vi "HEWH RLT PRAT.vi"() -> ()   [LabVIEW 2016] (continued)
            n244 = Bundle("Core"=T66 {"Current VI Reference"=refnum, "Close Panel on Exit?"=FALSE}, "DrawsLeft"=w600, "Error Log"=w599, "RLT Station Channels"="RLT Station Channels", "Station A Display"="Station A Display", "Station B Display"="Station B Display", "Station C Display"="Station C Display", "Station D Display"="Station D Display", "Draw Parameters Seq"=T41 {"Draws Left"=0, "Draws Left Array"=[], "Remaining Draws (A)"=1000, "Remaining Draws (B)"=1000, "Remaining Draws (C)"=1000, "Remaining Draws (D)"=1000, "Index of Element (A-D)"=[], "Station A"={"Sequence #"=0.0, "Cycles"=0, "Mode Setting"="", "Flow Rate (GPM)"=0.0, "Temperature (F)"=0.0, "Reset Timer"=FALSE, "Use Temp Decline Method"=FALSE, "Terminate Condition"=enum."C1-Terminate Draw @ Gallon Mark", "Condition Value #1"=0.0, "UE"=FALSE, "LE"=FALSE, "Comp"=FALSE, "Fan"=FALSE, "Test End Time (Sec)"=0.0, "Purge Until Cutout"=FALSE, "Start Conditions"=enum."Heat Source Cutout", "Condition Value #2"=0.0, "Remove Power"=FALSE, "Time"=0.0, "Check Special Cond."=enum."SC2-Check Heat Source (On-C2/Off-C1)", "Condition#"=enum."C1", "Draw Flags"=enum."N/A", "Data Processing Delay (FHD 15sec, UEF 5 Sec)"=0.0, "Test Complete"=FALSE}, "Station B"={"Sequence #"=0.0, "Cycles"=0, "Mode Setting"="", "Flow Rate (GPM)"=0.0, "Temperature (F)"=0.0, "Reset Timer"=FALSE, "Use Temp Decline Method"=FALSE, "Terminate Condition"=enum."C1-Terminate Draw @ Gallon Mark", "Condition Value #1"=0.0, "UE"=FALSE, "LE"=FALSE, "Comp"=FALSE, "Fan"=FALSE, "Test End Time (Sec)"=0.0, "Purge Until Cutout"=FALSE, "Start Conditions"=enum."Heat Source Cutout", "Condition Value #2"=0.0, "Remove Power"=FALSE, "Time"=0.0, "Check Special Cond."=enum."SC2-Check Heat Source (On-C2/Off-C1)", "Condition#"=enum."C1", "Draw Flags"=enum."N/A", "Data Processing Delay (FHD 15sec, UEF 5 Sec)"=0.0, "Test Complete"=FALSE}, "Station C"={"Sequence #"=0.0, "Cycles"=0, "Mode Setting"="", "Flow Rate (GPM)"=0.0, "Temperature (F)"=0.0, "Reset Timer"=FALSE, "Use Temp Decline Method"=FALSE, "Terminate Condition"=enum."C1-Terminate Draw @ Gallon Mark", "Condition Value #1"=0.0, "UE"=FALSE, "LE"=FALSE, "Comp"=FALSE, "Fan"=FALSE, "Test End Time (Sec)"=0.0, "Purge Until Cutout"=FALSE, "Start Conditions"=enum."Heat Source Cutout", "Condition Value #2"=0.0, "Remove Power"=FALSE, "Time"=0.0, "Check Special Cond."=enum."SC2-Check Heat Source (On-C2/Off-C1)", "Condition#"=enum."C1", "Draw Flags"=enum."N/A", "Data Processing Delay (FHD 15sec, UEF 5 Sec)"=0.0, "Test Complete"=FALSE}, "Station D"={"Sequence #"=0.0, "Cycles"=0, "Mode Setting"="", "Flow Rate (GPM)"=0.0, "Temperature (F)"=0.0, "Reset Timer"=FALSE, "Use Temp Decline Method"=FALSE, "Terminate Condition"=enum."C1-Terminate Draw @ Gallon Mark", "Condition Value #1"=0.0, "UE"=FALSE, "LE"=FALSE, "Comp"=FALSE, "Fan"=FALSE, "Test End Time (Sec)"=0.0, "Purge Until Cutout"=FALSE, "Start Conditions"=enum."Heat Source Cutout", "Condition Value #2"=0.0, "Remove Power"=FALSE, "Time"=0.0, "Check Special Cond."=enum."SC2-Check Heat Source (On-C2/Off-C1)", "Condition#"=enum."C1", "Draw Flags"=enum."N/A", "Data Processing Delay (FHD 15sec, UEF 5 Sec)"=0.0, "Test Complete"=FALSE}}, "Current Cond A"=w591, "Current Cond B"=w590, "Current Cond C"=w589, "Current Cond D"=w588, "Power Analyzer"=w587) -> (w597:T70)  [unwired: 1 in]
          }
        }
        n245 = call <vilib>:"Add State(s) to Queue__jki_lib_state_machine.vi"("State(s) in (\"\")"=w586) -> ("States Out"=w585:string)  [unwired: 14 in]
      }
      frame "Data: Cleanup" {
        n246 = Unbundle By Name(w606) -> ("Core.Current VI Reference"=w605:refnum<vi>)
        n247 = Close Reference(reference=w605, error in (no error)=w604) -> (error out=w602:errorcluster)
        n248 = call <vilib>:"Add State(s) to Queue__jki_lib_state_machine.vi"("State(s) in (\"\")"=w608) -> ("States Out"=w607:string)  [unwired: 14 in]
      }
      frame "---------- UI ----------" {
        n249 = call <vilib>:"Add State(s) to Queue__jki_lib_state_machine.vi"("State(s) in (\"\")"=w613) -> ("States Out"=w612:string)  [unwired: 14 in]
      }
      frame "UI: Initialize" {
        w617 = FALSE ("Recording Data")
        n250 = local write "Init Complete"(w617) -> ()
        n251 = local write "Alarm A"(w617) -> ()
        n252 = local write "Alarm B"(w617) -> ()
        n253 = local write "Alarm C"(w617) -> ()
        n254 = local write "Alarm D"(w617) -> ()
        n255 = property on="Start/Pause test" class="Bool (strict)"("DisabledEnum"=T67."Disabled and Grayed Out" ("Disabled")) -> ()  [unwired: 2 in, 2 out]
        n256 = local read "LV Program"() -> (w615:T24)
        n257 = case shown="\"PRAT\"" w615 {
          frame "HEWH", Default {
            w625 = T67."Disabled and Grayed Out" ("Disabled")
            w638 = T67."Disabled and Grayed Out" ("Disabled")
            w639 = HEWH_RLT_Station_Disable."Disable Station (No Draw)" ("Disable Station 2")
            w640 = T67."Disabled and Grayed Out" ("Disabled")
            w643 = FALSE ("DAQ for B")
            w644 = T67."Disabled and Grayed Out" ("Disabled")
            w627 = T67."Disabled and Grayed Out" ("Disabled")
            w632 = T67."Disabled and Grayed Out" ("Disabled")
            w645 = T67."Enabled" ("Disabled")
            n258 = property on="IF Start" class="Bool"("DisabledEnum"=w645) -> ()  [unwired: 2 in, 2 out]
            n259 = property on="Inlet Valve A" class="CmbBox (strict)"("DisabledEnum"=T67."Enabled" ("Disabled")) -> (error out=w633:errorcluster)  [unwired: 2 in, 1 out]
            n260 = property on="Drain Valve A" class="CmbBox (strict)"("DisabledEnum"=T67."Enabled" ("Disabled")) -> (error out=w630:errorcluster)  [unwired: 2 in, 1 out]
            n261 = property on="Outlet Valve A" class="CmbBox (strict)"("DisabledEnum"=T67."Enabled" ("Disabled")) -> (error out=w624:errorcluster)  [unwired: 2 in, 1 out]
            n262 = property on="DAQ for A" class="Bool (strict)"("DisabledEnum"=T67."Enabled" ("Disabled")) -> ()  [unwired: 2 in, 2 out]
            n263 = property on="DAQ for B" class="Bool (strict)"("DisabledEnum"=w644) -> ()  [unwired: 2 in, 2 out]
            n264 = property on="Inlet Valve B" class="CmbBox (strict)"(error in=w633, "DisabledEnum"=w632) -> (error out=w635:errorcluster)  [unwired: 1 in, 1 out]
            n265 = property on="Drain Valve B" class="CmbBox (strict)"(error in=w630, "DisabledEnum"=w627) -> (error out=w629:errorcluster)  [unwired: 1 in, 1 out]
            n266 = property on="Outlet Valve B" class="CmbBox (strict)"(error in=w624, "DisabledEnum"=w625) -> (error out=w623:errorcluster)  [unwired: 1 in, 1 out]
            n267 = property on="IF Stop" class="Bool"("DisabledEnum"=w645) -> ()  [unwired: 2 in, 2 out]
            n268 = property on="DAQ for C" class="Bool (strict)"("DisabledEnum"=w644) -> ()  [unwired: 2 in, 2 out]
            n269 = property on="Inlet Valve C" class="CmbBox (strict)"(error in=w635, "DisabledEnum"=w632) -> (error out=w634:errorcluster)  [unwired: 1 in, 1 out]
            n270 = property on="Drain Valve C" class="CmbBox (strict)"(error in=w629, "DisabledEnum"=w627) -> (error out=w628:errorcluster)  [unwired: 1 in, 1 out]
            n271 = property on="Outlet Valve C" class="CmbBox (strict)"(error in=w623, "DisabledEnum"=w625) -> (error out=w622:errorcluster)  [unwired: 1 in, 1 out]
            n272 = property on="HEWH Power" class="Bool (strict)"("DisabledEnum"=w645) -> ()  [unwired: 2 in, 2 out]
            n273 = property on="DAQ for D" class="Bool (strict)"("DisabledEnum"=w644) -> ()  [unwired: 2 in, 2 out]
            n274 = property on="Inlet Valve D" class="CmbBox (strict)"(error in=w634, "DisabledEnum"=w632) -> ()  [unwired: 1 in, 2 out]
            n275 = property on="Drain Valve D" class="CmbBox (strict)"(error in=w628, "DisabledEnum"=w627) -> ()  [unwired: 1 in, 2 out]
            n276 = property on="Outlet Valve D" class="CmbBox (strict)"(error in=w622, "DisabledEnum"=w625) -> ()  [unwired: 1 in, 2 out]
            n277 = property on="Disable Station 2" class="Enum (strict)"("Value"=w639) -> ()  [unwired: 2 in, 2 out]
            n278 = property on="Disable Station 3" class="Enum (strict)"("Value"=w639) -> ()  [unwired: 2 in, 2 out]
            n279 = property on="Disable Station 4" class="Enum (strict)"("Value"=w639) -> ()  [unwired: 2 in, 2 out]
            n280 = property on="Trigger Draw B" class="Bool"("DisabledEnum"=w638) -> ()  [unwired: 2 in, 2 out]
            n281 = property on="Trigger Draw C" class="Bool"("DisabledEnum"=w638) -> ()  [unwired: 2 in, 2 out]
            n282 = property on="Trigger Draw D" class="Bool"("DisabledEnum"=w638) -> ()  [unwired: 2 in, 2 out]
            n283 = property on="Disable Station 1" class="Enum (strict)"("DisabledEnum"=T67."Enabled" ("Disabled")) -> ()  [unwired: 2 in, 2 out]
            n284 = property on="Disable Station 2" class="Enum (strict)"("DisabledEnum"=w640) -> ()  [unwired: 2 in, 2 out]
            n285 = property on="Disable Station 3" class="Enum (strict)"("DisabledEnum"=w640) -> ()  [unwired: 2 in, 2 out]
            n286 = property on="Disable Station 4" class="Enum (strict)"("DisabledEnum"=w640) -> ()  [unwired: 2 in, 2 out]
            n287 = property on="Trigger Draw A" class="Bool"("DisabledEnum"=T67."Enabled" ("Disabled")) -> ()  [unwired: 2 in, 2 out]
            n288 = local write "DAQ for A"(TRUE ("DAQ for A")) -> ()
            n289 = local write "DAQ for B"(w643) -> ()
            n290 = local write "DAQ for C"(w643) -> ()
            n291 = local write "DAQ for D"(w643) -> ()
          }
          frame "HEWH RLT" {
            w650 = T67."Enabled" ("Disabled")
            w652 = T67."Enabled" ("Disabled")
            w657 = T67."Enabled" ("Disabled")
            w662 = T67."Enabled" ("Disabled")
            w663 = T67."Enabled" ("Disabled")
            w664 = FALSE ("DAQ for B")
            w666 = T67."Enabled" ("Disabled")
            w665 = T67."Enabled" ("Disabled")
            n292 = property on="IF Start" class="Bool"("DisabledEnum"=w665) -> ()  [unwired: 2 in, 2 out]
            n293 = property on="Inlet Valve A" class="CmbBox (strict)"("DisabledEnum"=T67."Enabled" ("Disabled")) -> (error out=w658:errorcluster)  [unwired: 2 in, 1 out]
            n294 = property on="Drain Valve A" class="CmbBox (strict)"("DisabledEnum"=T67."Enabled" ("Disabled")) -> (error out=w655:errorcluster)  [unwired: 2 in, 1 out]
            n295 = property on="Outlet Valve A" class="CmbBox (strict)"("DisabledEnum"=T67."Enabled" ("Disabled")) -> (error out=w649:errorcluster)  [unwired: 2 in, 1 out]
            n296 = property on="DAQ for A" class="Bool (strict)"("DisabledEnum"=w666) -> ()  [unwired: 2 in, 2 out]
            n297 = property on="DAQ for B" class="Bool (strict)"("DisabledEnum"=w666) -> ()  [unwired: 2 in, 2 out]
            n298 = property on="Inlet Valve B" class="CmbBox (strict)"(error in=w658, "DisabledEnum"=w657) -> (error out=w660:errorcluster)  [unwired: 1 in, 1 out]
            n299 = property on="Drain Valve B" class="CmbBox (strict)"(error in=w655, "DisabledEnum"=w652) -> (error out=w654:errorcluster)  [unwired: 1 in, 1 out]
            n300 = property on="Outlet Valve B" class="CmbBox (strict)"(error in=w649, "DisabledEnum"=w650) -> (error out=w648:errorcluster)  [unwired: 1 in, 1 out]
            n301 = property on="IF Stop" class="Bool"("DisabledEnum"=w665) -> ()  [unwired: 2 in, 2 out]
            n302 = property on="DAQ for C" class="Bool (strict)"("DisabledEnum"=w666) -> ()  [unwired: 2 in, 2 out]
            n303 = property on="Inlet Valve C" class="CmbBox (strict)"(error in=w660, "DisabledEnum"=w657) -> (error out=w659:errorcluster)  [unwired: 1 in, 1 out]
            n304 = property on="Drain Valve C" class="CmbBox (strict)"(error in=w654, "DisabledEnum"=w652) -> (error out=w653:errorcluster)  [unwired: 1 in, 1 out]
            n305 = property on="Outlet Valve C" class="CmbBox (strict)"(error in=w648, "DisabledEnum"=w650) -> (error out=w647:errorcluster)  [unwired: 1 in, 1 out]
            n306 = property on="HEWH Power" class="Bool (strict)"("DisabledEnum"=w665) -> ()  [unwired: 2 in, 2 out]
            n307 = property on="DAQ for D" class="Bool (strict)"("DisabledEnum"=w666) -> ()  [unwired: 2 in, 2 out]
            n308 = property on="Inlet Valve D" class="CmbBox (strict)"(error in=w659, "DisabledEnum"=w657) -> ()  [unwired: 1 in, 2 out]
            n309 = property on="Drain Valve D" class="CmbBox (strict)"(error in=w653, "DisabledEnum"=w652) -> ()  [unwired: 1 in, 2 out]
            n310 = property on="Outlet Valve D" class="CmbBox (strict)"(error in=w647, "DisabledEnum"=w650) -> ()  [unwired: 1 in, 2 out]
            n311 = property on="Trigger Draw D" class="Bool"("DisabledEnum"=w662) -> ()  [unwired: 2 in, 2 out]
            n312 = property on="Trigger Draw C" class="Bool"("DisabledEnum"=w662) -> ()  [unwired: 2 in, 2 out]
            n313 = property on="Trigger Draw B" class="Bool"("DisabledEnum"=w662) -> ()  [unwired: 2 in, 2 out]
            n314 = property on="Trigger Draw A" class="Bool"("DisabledEnum"=w662) -> ()  [unwired: 2 in, 2 out]
            n315 = local write "DAQ for B"(w664) -> ()
            n316 = local write "DAQ for C"(w664) -> ()
            n317 = local write "DAQ for D"(w664) -> ()
            n318 = local write "DAQ for A"(w664) -> ()
            n319 = property on="Disable Station 1" class="Enum (strict)"("DisabledEnum"=w663) -> ()  [unwired: 2 in, 2 out]
            n320 = property on="Disable Station 2" class="Enum (strict)"("DisabledEnum"=w663) -> ()  [unwired: 2 in, 2 out]
            n321 = property on="Disable Station 3" class="Enum (strict)"("DisabledEnum"=w663) -> ()  [unwired: 2 in, 2 out]
            n322 = property on="Disable Station 4" class="Enum (strict)"("DisabledEnum"=w663) -> ()  [unwired: 2 in, 2 out]
          }
          frame "PRAT" {
            w670 = T67."Disabled and Grayed Out" ("Disabled")
            w672 = T67."Disabled and Grayed Out" ("Disabled")
            w677 = T67."Enabled" ("Disabled")
            w682 = T67."Enabled" ("Disabled")
            w683 = T67."Enabled" ("Disabled")
            w684 = FALSE ("DAQ for B")
            w686 = T67."Disabled and Grayed Out" ("Disabled")
            w685 = T67."Disabled and Grayed Out" ("Disabled")
            n323 = property on="Trigger Draw A" class="Bool"("DisabledEnum"=w682) -> ()  [unwired: 2 in, 2 out]
            n324 = property on="DAQ for A" class="Bool (strict)"("DisabledEnum"=w686) -> ()  [unwired: 2 in, 2 out]
            n325 = property on="IF Start" class="Bool"("DisabledEnum"=w685) -> ()  [unwired: 2 in, 2 out]
            n326 = property on="Trigger Draw B" class="Bool"("DisabledEnum"=w682) -> ()  [unwired: 2 in, 2 out]
            n327 = property on="Inlet Valve A" class="CmbBox (strict)"("DisabledEnum"=T67."Enabled" ("Disabled")) -> (error out=w678:errorcluster)  [unwired: 2 in, 1 out]
            n328 = property on="Drain Valve A" class="CmbBox (strict)"("DisabledEnum"=T67."Disabled and Grayed Out" ("Disabled")) -> (error out=w675:errorcluster)  [unwired: 2 in, 1 out]
            n329 = property on="Outlet Valve A" class="CmbBox (strict)"("DisabledEnum"=T67."Disabled and Grayed Out" ("Disabled")) -> (error out=w669:errorcluster)  [unwired: 2 in, 1 out]
            n330 = property on="DAQ for B" class="Bool (strict)"("DisabledEnum"=w686) -> ()  [unwired: 2 in, 2 out]
            n331 = property on="IF Stop" class="Bool"("DisabledEnum"=w685) -> ()  [unwired: 2 in, 2 out]
            n332 = property on="Trigger Draw C" class="Bool"("DisabledEnum"=w682) -> ()  [unwired: 2 in, 2 out]
            n333 = property on="DAQ for C" class="Bool (strict)"("DisabledEnum"=w686) -> ()  [unwired: 2 in, 2 out]
            n334 = property on="Inlet Valve B" class="CmbBox (strict)"(error in=w678, "DisabledEnum"=w677) -> (error out=w680:errorcluster)  [unwired: 1 in, 1 out]
            n335 = property on="Drain Valve B" class="CmbBox (strict)"(error in=w675, "DisabledEnum"=w672) -> (error out=w674:errorcluster)  [unwired: 1 in, 1 out]
            n336 = property on="Outlet Valve B" class="CmbBox (strict)"(error in=w669, "DisabledEnum"=w670) -> (error out=w668:errorcluster)  [unwired: 1 in, 1 out]
            n337 = property on="HEWH Power" class="Bool (strict)"("DisabledEnum"=w685) -> ()  [unwired: 2 in, 2 out]
            n338 = property on="DAQ for D" class="Bool (strict)"("DisabledEnum"=w686) -> ()  [unwired: 2 in, 2 out]
            n339 = property on="Trigger Draw D" class="Bool"("DisabledEnum"=w682) -> ()  [unwired: 2 in, 2 out]
            n340 = property on="Inlet Valve C" class="CmbBox (strict)"(error in=w680, "DisabledEnum"=w677) -> (error out=w679:errorcluster)  [unwired: 1 in, 1 out]
            n341 = property on="Drain Valve C" class="CmbBox (strict)"(error in=w674, "DisabledEnum"=w672) -> (error out=w673:errorcluster)  [unwired: 1 in, 1 out]
            n342 = property on="Outlet Valve C" class="CmbBox (strict)"(error in=w668, "DisabledEnum"=w670) -> (error out=w667:errorcluster)  [unwired: 1 in, 1 out]
            n343 = property on="Inlet Valve D" class="CmbBox (strict)"(error in=w679, "DisabledEnum"=w677) -> ()  [unwired: 1 in, 2 out]
            n344 = property on="Drain Valve D" class="CmbBox (strict)"(error in=w673, "DisabledEnum"=w672) -> ()  [unwired: 1 in, 2 out]
            n345 = property on="Outlet Valve D" class="CmbBox (strict)"(error in=w667, "DisabledEnum"=w670) -> ()  [unwired: 1 in, 2 out]
            n346 = local write "DAQ for B"(w684) -> ()
            n347 = local write "DAQ for C"(w684) -> ()
            n348 = local write "DAQ for D"(w684) -> ()
            n349 = local write "DAQ for A"(w684) -> ()
            n350 = property on="Disable Station 1" class="Enum (strict)"("DisabledEnum"=w683) -> ()  [unwired: 2 in, 2 out]
            n351 = property on="Disable Station 2" class="Enum (strict)"("DisabledEnum"=w683) -> ()  [unwired: 2 in, 2 out]
            n352 = property on="Disable Station 3" class="Enum (strict)"("DisabledEnum"=w683) -> ()  [unwired: 2 in, 2 out]
            n353 = property on="Disable Station 4" class="Enum (strict)"("DisabledEnum"=w683) -> ()  [unwired: 2 in, 2 out]
          }
        }
        n354 = call <vilib>:"Add State(s) to Queue__jki_lib_state_machine.vi"("State(s) in (\"\")"=w621) -> ("States Out"=w620:string)  [unwired: 14 in]
      }
      frame "UI: Cursor Set" {
        # "Argument"
        # "Set and Unset Cursor Busy.\n(Usage: \"UI: Cursor Set >> Busy|Idle\")"
        n355 = case shown="\"Busy\"" w688 {
          tunnel: w690 -> [w695 w697]
          tunnel: [w694 w696] -> w689
          frame "Idle", Default {
            n356 = call <vilib>:"Unset Busy.vi"("error in (no error)"=w695) -> ("error out"=w694:errorcluster)  [unwired: 10 in]
          }
          frame "Busy" {
            n357 = call <vilib>:"Set Busy.vi"("error in (no error)"=w697) -> ("error out"=w696:errorcluster)  [unwired: 9 in, 1 out]
          }
        }
        n358 = call <vilib>:"Add State(s) to Queue__jki_lib_state_machine.vi"("State(s) in (\"\")"=w693) -> ("States Out"=w692:string)  [unwired: 14 in]
      }
      frame "UI: Front Panel State" {
        # "Argument"
        n359 = Unbundle By Name(w701) -> ("Core.Current VI Reference"=w700:refnum<vi>)
        n360 = case shown="\"Open\", Default" w699 {
          tunnel: w703 -> [w709 w722]
          tunnel: [w711 w723] -> w702
          tunnel: w700 -> [w710 w720]
          frame "Open", Default {
            n361 = property class="VI"(reference=w710, error in=w709) -> (reference out=w707:refnum<vi>, error out=w708:errorcluster, "Front Panel.Open"=w706:bool)
            n362 = case shown="False" w706 {
              tunnel: [w714 w717] -> w711
              tunnel: w708 -> [w713 w717]
              tunnel: w707 -> [w712 _]
              frame False {
                n363 = invoke class="VI" method="FP.Open"(reference=w712, error in=w713, "Activate"=TRUE, "State"=T68."Maximized") -> (error out=w714:errorcluster)  [unwired: 1 in, 4 out]
              }
              frame True {
              }
            }
          }
          frame "Close" {
            n364 = property class="VI"(reference=w720, error in=w722) -> (reference out=w719:refnum<vi>, error out=w721:errorcluster, "Front Panel.Open"=w718:bool)
            n365 = case shown="False" w718 {
              tunnel: [w724 w727] -> w723
              tunnel: w721 -> [w724 w726]
              tunnel: w719 -> [_ w725]
              frame False {
              }
              frame True {
                n366 = disable-structure shown="Enabled" {
                  disable-tunnel: [w730 w731] -> w727
                  disable-tunnel: w726 -> [w729 w731]
                  disable-tunnel: w725 -> [w728 _]
                  frame Disabled {
                    n367 = invoke class="VI" method="FP.Close"(reference=w728, error in=w729) -> (error out=w730:errorcluster)  [unwired: 1 in, 2 out]
                  }
                  frame Enabled {
                  }
                }
              }
            }
          }
        }
        n368 = call <vilib>:"Add State(s) to Queue__jki_lib_state_machine.vi"("State(s) in (\"\")"=w705) -> ("States Out"=w704:string)  [unwired: 14 in]
      }
      frame "---------- Macro ----------" {
        n369 = call <vilib>:"Add State(s) to Queue__jki_lib_state_machine.vi"("State(s) in (\"\")"=w736) -> ("States Out"=w735:string)  [unwired: 14 in]
      }
      frame "Macro: Initialize" {
        w738 = "Data: Initialize\nInitialize Core Data\nUI: Initialize\nUI: Front Panel State >> Open\nInitialize Channels\nInitialize Files\nTest: Update Display A\nTest: Update Display B\nTest: Update Display C\nTest: Update Display D\nInit Complete"  # Data: Initialize Initialize Core Data UI: Initialize UI: Front Panel State >> Open Initialize Channels Initialize Files Test: Update Display A Test: Update Display B Test: Update Display C Test: Update Display D Init Complete
        n370 = call <vilib>:"Add State(s) to Queue__jki_lib_state_machine.vi"("State(s) in Front (\"\")"=w738, "State(s) in (\"\")"=w742) -> ("States Out"=w741:string)  [unwired: 13 in]
      }
      frame "Macro: Exit" {
        n371 = Unbundle By Name(w750) -> ("Core.Close Panel on Exit?"=w749:bool)
        n372 = Select(t="UI: Front Panel State >> Close", s=w749, f="") -> (s? t:f=w746:string)
        n373 = call <vilib>:"Add State(s) to Queue__jki_lib_state_machine.vi"("State(s) in (\"\")"=w746, "State(s) at Back (\"\")"="Data: Cleanup\nExit") -> ("States Out"=w744:string)  [unwired: 13 in]
        n374 = call <vilib>:"Add State(s) to Queue__jki_lib_state_machine.vi"("State(s) in Front (\"\")"=w744, "State(s) in (\"\")"=w753) -> ("States Out"=w752:string)  [unwired: 13 in]
      }
      frame "---------- Test ----------" {
        n375 = call <vilib>:"Add State(s) to Queue__jki_lib_state_machine.vi"("State(s) in (\"\")"=w758) -> ("States Out"=w757:string)  [unwired: 14 in]
      }
      frame "Test: Check Complete" {
        n376 = Unbundle By Name(w788) -> ("Station A Display.Display Data (RLT).Cycle Count Display"=w780:i32, "Station A Display.Display Data (RLT).Cycle Count Display"=w781:i32, "Station A Display.Display Data (RLT).Cycle Count Display"=w782:i32, "Station A Display.Display Data (RLT).Cycle Count Display"=w783:i32)
        n377 = local read "Station A Test Sequence"() -> (w787:T14[])
        n378 = local read "Station B Test Sequence"() -> (w786:T14[])
        n379 = local read "Station C Test Sequence"() -> (w785:T14[])
        n380 = local read "Station D Test Sequence"() -> (w784:T14[])
        n381 = local read "Use Last Start Condition A?"() -> (w774:bool)
        n382 = local read "Use Last Start Condition B?"() -> (w773:bool)
        n383 = local read "Use Last Start Condition C?"() -> (w772:bool)
        n384 = local read "Use Last Start Condition D?"() -> (w771:bool)
        n385 = call "PRAT Multi Station Check.vi"("Station A Test Sequence"=w787, "Station B Test Sequence"=w786, "Station C Test Sequence"=w785, "Station D Test Sequence"=w784, "Error In"=w779, "Cycle Count Display (Station A)"=w783, "Use Last Start Condition A?"=w774, "Cycle Count Display (Station B)"=w782, "Cycle Count Display (Station C)"=w781, "Use Last Start Condition B?"=w773, "Cycle Count Display (Station D)"=w780, "Use Last Start Condition C?"=w772, "Use Last Start Condition D?"=w771) -> ("Draw Parameters"=w770:T41, "Error Out"=w761:errorcluster)  [unwired: 13 in]
        "Current Draw Parameters" <- w770
        n386 = Unbundle By Name(w770) -> ("Remaining Draws (A)"=→"Remaining Draws (A)":i32, "Remaining Draws (B)"=→"Remaining Draws (B)":i32, "Remaining Draws (C)"=→"Remaining Draws (C)":i32, "Remaining Draws (D)"=→"Remaining Draws (D)":i32, "Draws Left"=w769:i32)
        "Draws Left" <- w769
        n387 = local read "Log Data Output (D)"() -> (w766:bool)
        n388 = local read "Log Data Output (C)"() -> (w765:bool)
        n389 = local read "LV Program"() -> (w762:T24)
        n390 = local read "Log Data Output (A)"() -> (w768:bool)
        n391 = local read "Log Data Output (B)"() -> (w767:bool)
        n392 = call "HEWH Create Save Data States.vi"("LV Program"=w762, "Data Loop?"=FALSE, "Error In"=w761, "Log Data Output (C)"=w765, "Log Data Output (A)"=w768, "Log Data Output (D)"=w766, "Log Data Output (B)"=w767) -> ("SM States"=w763:string, "Error Out"=w760:errorcluster)  [unwired: 11 in]
        n393 = case shown="0" w769 {
          tunnel: w760 -> [w794 w798]
          tunnel: [w793 w798] -> w759
          frame 0 {
            n394 = call "UTILITY String Notifier.vi"("Status"=UTILITY_Notifier."Set", "error in (no error)"=w794, "Set Status"=T7 "All Draws Complete..." ("Message"), "name (unnamed)"="Message") -> ("error out"=w793:errorcluster)  [unwired: 6 in, 1 out]
          }
          frame 1, Default {
          }
        }
        n395 = Bundle By Name(cluster=w788, "Draw Parameters Seq"=w770) -> (w790:T70)
        n396 = call <vilib>:"Add State(s) to Queue__jki_lib_state_machine.vi"("State(s) in Front (\"\")"=w763, "State(s) in (\"\")"=w792) -> ("States Out"=w791:string)  [unwired: 13 in]
      }
      frame "Test: Update Display A" {
        n397 = local read "Appliance Details A"() -> (w799:T4)
        n398 = local read "Current (A)"() -> (w808:dbl)
        n399 = Bundle By Name(cluster=w809, "Station A Display.Display Data (RLT).Current Display"=w808, "Station A Display.Appliance Details"=w799) -> (w807:T70)
        n400 = Unbundle By Name(w807) -> ("Station A Display.Display Data (RLT).Station Label Display"=w805:string, "Station A Display.Display Data (RLT).Board ID Display"=w804:string, "Station A Display.Display Data (RLT).Serial Number Display"=w803:string, "Station A Display.Display Data (RLT).Current Display"=w802:dbl, "Station A Display.Display Data (RLT).Status Color"=w801:u32, "Station A Display.Display Data (RLT).Cycle Count Display"=w800:i32)
        n401 = property on="Station Label Display" class="Str"("Value"=w805) -> ()  [unwired: 2 in, 2 out]
        n402 = property on="Board ID Display" class="Str"("Value"=w804) -> ()  [unwired: 2 in, 2 out]
        n403 = property on="Serial Number Display" class="Str"("Value"=w803) -> ()  [unwired: 2 in, 2 out]
        n404 = property on="Current Display" class="DigNum (strict)"("Value"=w802) -> ()  [unwired: 2 in, 2 out]
        n405 = property on="Status Color" class="ColBox"("Value"=w801) -> ()  [unwired: 2 in, 2 out]
        n406 = property on="Cycle Count Display" class="DigNum (strict)"("Value"=w800) -> ()  [unwired: 2 in, 2 out]
        n407 = call <vilib>:"Add State(s) to Queue__jki_lib_state_machine.vi"("State(s) in (\"\")"=w812) -> ("States Out"=w811:string)  [unwired: 14 in]
      }
      frame "Test: Update Display B" {
        n408 = local read "Appliance Details B"() -> (w813:T4)
        n409 = local read "Current (B)"() -> (w822:dbl)
        n410 = Bundle By Name(cluster=w823, "Station B Display.Display Data (RLT).Current Display"=w822, "Station B Display.Appliance Details"=w813) -> (w821:T70)
        n411 = Unbundle By Name(w821) -> ("Station B Display.Display Data (RLT).Station Label Display"=w819:string, "Station B Display.Display Data (RLT).Board ID Display"=w818:string, "Station B Display.Display Data (RLT).Serial Number Display"=w817:string, "Station B Display.Display Data (RLT).Current Display"=w816:dbl, "Station B Display.Display Data (RLT).Status Color"=w815:u32, "Station B Display.Display Data (RLT).Cycle Count Display"=w814:i32)
        n412 = property on="Cycle Count Display" class="DigNum (strict)"("Value"=w814) -> ()  [unwired: 2 in, 2 out]
        n413 = property on="Current Display" class="DigNum (strict)"("Value"=w816) -> ()  [unwired: 2 in, 2 out]
        n414 = property on="Station Label Display" class="Str"("Value"=w819) -> ()  [unwired: 2 in, 2 out]
        n415 = property on="Board ID Display" class="Str"("Value"=w818) -> ()  [unwired: 2 in, 2 out]
        n416 = property on="Serial Number Display" class="Str"("Value"=w817) -> ()  [unwired: 2 in, 2 out]
        n417 = property on="Status Color" class="ColBox"("Value"=w815) -> ()  [unwired: 2 in, 2 out]
        n418 = call <vilib>:"Add State(s) to Queue__jki_lib_state_machine.vi"("State(s) in (\"\")"=w826) -> ("States Out"=w825:string)  [unwired: 14 in]
      }
      frame "Test: Update Display C" {
        n419 = local read "Appliance Details C"() -> (w827:T4)
        n420 = local read "Current (C)"() -> (w836:dbl)
        n421 = Bundle By Name(cluster=w837, "Station C Display.Display Data (RLT).Current Display"=w836, "Station C Display.Appliance Details"=w827) -> (w835:T70)
        n422 = Unbundle By Name(w835) -> ("Station C Display.Display Data (RLT).Station Label Display"=w833:string, "Station C Display.Display Data (RLT).Board ID Display"=w832:string, "Station C Display.Display Data (RLT).Serial Number Display"=w831:string, "Station C Display.Display Data (RLT).Current Display"=w830:dbl, "Station C Display.Display Data (RLT).Status Color"=w829:u32, "Station C Display.Display Data (RLT).Cycle Count Display"=w828:i32)
        n423 = property on="Station Label Display" class="Str"("Value"=w833) -> ()  [unwired: 2 in, 2 out]
        n424 = property on="Board ID Display" class="Str"("Value"=w832) -> ()  [unwired: 2 in, 2 out]
        n425 = property on="Serial Number Display" class="Str"("Value"=w831) -> ()  [unwired: 2 in, 2 out]
        n426 = property on="Current Display" class="DigNum (strict)"("Value"=w830) -> ()  [unwired: 2 in, 2 out]
        n427 = property on="Status Color" class="ColBox"("Value"=w829) -> ()  [unwired: 2 in, 2 out]
        n428 = property on="Cycle Count Display" class="DigNum (strict)"("Value"=w828) -> ()  [unwired: 2 in, 2 out]
        n429 = call <vilib>:"Add State(s) to Queue__jki_lib_state_machine.vi"("State(s) in (\"\")"=w840) -> ("States Out"=w839:string)  [unwired: 14 in]
      }
      frame "Test: Update Display D" {
        n430 = local read "Appliance Details D"() -> (w841:T4)
        n431 = local read "Current (D)"() -> (w850:dbl)
        n432 = Bundle By Name(cluster=w851, "Station D Display.Display Data (RLT).Current Display"=w850, "Station D Display.Appliance Details"=w841) -> (w849:T70)
        n433 = Unbundle By Name(w849) -> ("Station D Display.Display Data (RLT).Station Label Display"=w847:string, "Station D Display.Display Data (RLT).Board ID Display"=w846:string, "Station D Display.Display Data (RLT).Serial Number Display"=w845:string, "Station D Display.Display Data (RLT).Current Display"=w844:dbl, "Station D Display.Display Data (RLT).Status Color"=w843:u32, "Station D Display.Display Data (RLT).Cycle Count Display"=w842:i32)
        n434 = property on="Station Label Display" class="Str"("Value"=w847) -> ()  [unwired: 2 in, 2 out]
        n435 = property on="Board ID Display" class="Str"("Value"=w846) -> ()  [unwired: 2 in, 2 out]
        n436 = property on="Serial Number Display" class="Str"("Value"=w845) -> ()  [unwired: 2 in, 2 out]
        n437 = property on="Current Display" class="DigNum (strict)"("Value"=w844) -> ()  [unwired: 2 in, 2 out]
        n438 = property on="Status Color" class="ColBox"("Value"=w843) -> ()  [unwired: 2 in, 2 out]
        n439 = property on="Cycle Count Display" class="DigNum (strict)"("Value"=w842) -> ()  [unwired: 2 in, 2 out]
        n440 = call <vilib>:"Add State(s) to Queue__jki_lib_state_machine.vi"("State(s) in (\"\")"=w854) -> ("States Out"=w853:string)  [unwired: 14 in]
      }
      frame "Test: Wait for Power Off (Station A)" {
        # "I should use an event to change the condition value...its just more wires/\ncomplications...not sure its worth it."
        # "Need to add final conditions\nfor both 24hr and 1hr"
        n441 = Unbundle By Name(w899) -> ("Station A Display.Display Data (RLT)"=w890:T29, "Draw Parameters Seq"=w888:T41, "Current Cond A"=w881:T1, "Draw Parameters Seq.Station A.Reset Timer"=w856:bool)
        n442 = local read "Core HEWH Data Input A"() -> (w883:T12)
        n443 = call "HEWH Station Timer.vi"("Station ID"=Station_ID_Selector."A", "error in (no error)"=w855, "Reset Timer (A)"="Reset Timer (A)", "Reset Timer (Cluster)"=w856) -> ("error out"=w861:errorcluster, "Elapsed Time (sec)- String"=w857:string, "Elapsed Time (sec)"=w859:dbl)  [unwired: 5 in]
        "A Timer" <- w859
        n444 = Format Date/Time String(time format string (%c)="%H:%M:%S%3u", seconds (now)=w859, UTC format=TRUE) -> (date/time string=→"Timer 1":string)
        n445 = local read "Purge Time (Seconds)"() -> (w858:dbl)
        n446 = local read "Draw Station"() -> (w891:string)
        n447 = local read "Start Draw"() -> (w894:bool)
        n448 = Bundle By Name(cluster=w883, "Current Cond"=w881) -> (w882:T12)
        n449 = call "UTILITY String Notifier.vi"("Status"=UTILITY_Notifier."Set", "error in (no error)"=w861, "Set Status"=w857, "name (unnamed)"="TimerA") -> ("error out"=w860:errorcluster)  [unwired: 6 in, 1 out]
        n450 = call "HEWH Conditional Trigger.vi"("Draw Parameters Seq"=w888, "Core HEWH Data Input"=w882, "Station"="A", "Manual Draw Trigger"="Trigger Draw A", "Draw Station"=w891, "Error In"=w860, "Start Draw"=w894, "Purge Time (sec)"=w858, "Delay After Cutout (sec)"="Cutout Delay A (sec)", "A Timer"=w859, "Disable Station in"="Disable Station 1", "StationA Setpoint"="StationA Setpoint", "Display Data (RLT) In"=w890) -> ("Station Data Output"=w864:T14, "Use Last Start Condition?"=→"Use Last Start Condition A?":bool, "SM States"=w893:string, "Display Data (RLT) Out"=w871:T29, "Core HEWH Data Output"=w874:T12, "Disable Station"=w878:bool, "Error Out"=w884:errorcluster)  [unwired: 7 in, 1 out]
        n451 = Unbundle By Name(w874) -> ("Test Complete"=w873:bool)
        "Test CompleteA" <- w873
        n452 = Unbundle By Name(w874) -> ("Current Cond"=w880:T1)
        "Condition A" <- w880
        n453 = call "HEWH End Of Test Display.vi"("String Notifier"="MessageA", "error in (no error)"=w884, "Disable Station"=w878, "Current Cond"=w880) -> ("error out"=w876:errorcluster, "Failure"=w872:bool)  [unwired: 6 in]
        n454 = Or(x=w878, y=w872) -> (x .or. y?=w877:bool)
        n455 = local read "HEWH Power"() -> (w867:bool)
        n456 = case shown="True" w877 {
          tunnel: w876 -> [w909 w914]
          tunnel: [w909 w913] -> w875
          tunnel: w873 -> [_ w912]
          tunnel: w872 -> [_ w911]
          frame False {
          }
          frame True {
            n457 = Or(x=w912, y=w911) -> (x .or. y?=w910:bool)
            n458 = case shown="True" w910 {
              tunnel: w914 -> [w916 w919]
              tunnel: [w916 w918] -> w913
              frame False {
              }
              frame True {
                n459 = flat-sequence {
                  tunnel: w919 -> [w922]
                  tunnel: [w922] -> w917
                  tunnel: [w924] -> w918
                  tunnel: w917 -> [w924]
                  frame #0 {
                    n460 = local write "Log Data Output (A)"(FALSE ("Log Data Output (A)")) -> ()
                    n461 = local write "Station ID to Reset"(Station_ID_Selector."A" ("Station ID to Reset")) -> ()
                  }
                  frame #1 {
                    "Final Headers A" <- TRUE ("Final Headers A")
                  }
                }
              }
            }
            n462 = local write "Disable Station 1"(HEWH_RLT_Station_Disable."Disable Station (No Draw)" ("Disable Station 1")) -> ()
          }
        }
        n463 = Bundle By Name(cluster=w899, "Station A Display.Display Data (RLT)"=w871, "Current Cond A"=w880) -> (w898:T70)
        n464 = call "HEWH Check Power Set.vi"("Station Data Output"=w864, "Timer"=w859, "HEWH Power"=w867) -> ("Set Power To This Value"=w865:bool, "Trigger Power Set"=w866:bool)  [unwired: 6 in, 1 out]
        n465 = case shown="True" w866 {
          tunnel: w865 -> [_ w906]
          frame False {
          }
          frame True {
            n466 = property on="HEWH Power" class="Bool (strict)"("Val(Sgnl)"=w906) -> ()  [unwired: 2 in, 2 out]
            n467 = case shown="False" w906 {
              tunnel: ["Power OFF..." ("Set Status") "Power ON..." ("Set Status")] -> w903
              frame False {
              }
              frame True {
              }
            }
            n468 = call "UTILITY String Notifier.vi"("Status"=UTILITY_Notifier."Set", "Set Status"=w903, "name (unnamed)"="MessageA") -> ()  [unwired: 7 in, 2 out]
          }
        }
        n469 = call <vilib>:"Add State(s) to Queue__jki_lib_state_machine.vi"("State(s) in Front (\"\")"=w893, "State(s) in (\"\")"=w902) -> ("States Out"=w901:string)  [unwired: 13 in]
      }
      frame "Test: Wait for Power Off (Station B)" {
        # "B Timer"
        # "Main Test Loop: Decides which Tank to Run, and starts that sequence."
        n470 = Unbundle By Name(w969) -> ("Station B Display.Display Data (RLT)"=w959:T29, "Draw Parameters Seq"=w966:T41, "Current Cond B"=w951:T1, "Draw Parameters Seq.Station B.Reset Timer"=w926:bool)
        n471 = local read "Core HEWH Data Input B"() -> (w953:T12)
        n472 = Bundle By Name(cluster=w953, "Current Cond"=w951) -> (w952:T12)
        n473 = call "HEWH Station Timer.vi"("Station ID"=Station_ID_Selector."B", "error in (no error)"=w925, "Reset Timer (A)"="Reset Timer (B)", "Reset Timer (Cluster)"=w926) -> ("error out"=w931:errorcluster, "Elapsed Time (sec)- String"=w927:string, "Elapsed Time (sec)"=w929:dbl)  [unwired: 5 in]
        "B Timer" <- w929
        n474 = call "UTILITY String Notifier.vi"("Status"=UTILITY_Notifier."Set", "error in (no error)"=w931, "Set Status"=w927, "name (unnamed)"="TimerB") -> ("error out"=w930:errorcluster)  [unwired: 6 in, 1 out]
        n475 = local read "Purge Time (Seconds)"() -> (w928:dbl)
        n476 = local read "Draw Station"() -> (w960:string)
        n477 = local read "Start Draw"() -> (w963:bool)
        n478 = call "HEWH Conditional Trigger.vi"("Draw Parameters Seq"=w966, "Core HEWH Data Input"=w952, "Station"="B", "Manual Draw Trigger"="Trigger Draw B", "Draw Station"=w960, "Error In"=w930, "Start Draw"=w963, "Purge Time (sec)"=w928, "Delay After Cutout (sec)"="Cutout Delay B (sec)", "A Timer"=w929, "Disable Station in"="Disable Station 2", "StationA Setpoint"="StationB Setpoint", "Display Data (RLT) In"=w959) -> ("Station Data Output"=w934:T14, "Use Last Start Condition?"=→"Use Last Start Condition B?":bool, "SM States"=w962:string, "Display Data (RLT) Out"=w958:T29, "Core HEWH Data Output"=w943:T12, "Disable Station"=w947:bool, "Error Out"=w949:errorcluster)  [unwired: 7 in, 1 out]
        n479 = Format Date/Time String(time format string (%c)="%H:%M:%S%3u", seconds (now)=w929, UTC format=TRUE) -> (date/time string=→"Timer 2":string)
        n480 = Unbundle By Name(w943) -> ("Test Complete"=w942:bool)
        "Test CompleteB" <- w942
        n481 = Unbundle By Name(w943) -> ("Current Cond"=w950:T1)
        "Condition B" <- w950
        n482 = call "HEWH End Of Test Display.vi"("String Notifier"="MessageB" ("name (unnamed)"), "error in (no error)"=w949, "Disable Station"=w947, "Current Cond"=w950) -> ("error out"=w945:errorcluster, "Failure"=w941:bool)  [unwired: 6 in]
        n483 = Or(x=w941, y=w947) -> (x .or. y?=w946:bool)
        n484 = case shown="True" w946 {
          tunnel: w945 -> [w979 w984]
          tunnel: [w979 w983] -> w944
          tunnel: w942 -> [_ w982]
          tunnel: w941 -> [_ w980]
          frame False {
          }
          frame True {
            n485 = Or(x=w982, y=w980) -> (x .or. y?=w981:bool)
            n486 = case shown="True" w981 {
              tunnel: w984 -> [w986 w989]
              tunnel: [w986 w988] -> w983
              frame False {
              }
              frame True {
                n487 = flat-sequence {
                  tunnel: w989 -> [w992]
                  tunnel: [w992] -> w987
                  tunnel: [w994] -> w988
                  tunnel: w987 -> [w994]
                  frame #0 {
                    n488 = local write "Log Data Output (B)"(FALSE ("Log Data Output (A)")) -> ()
                    n489 = local write "Station ID to Reset"(Station_ID_Selector."B" ("Station ID to Reset")) -> ()
                  }
                  frame #1 {
                    "Final Headers B" <- TRUE ("Final Headers B")
                  }
                }
              }
            }
            n490 = local write "Disable Station 2"(HEWH_RLT_Station_Disable."Disable Station (No Draw)" ("Disable Station 1")) -> ()
          }
        }
        n491 = local read "HEWH Power"() -> (w938:bool)
        n492 = Bundle By Name(cluster=w969, "Station B Display.Display Data (RLT)"=w958, "Current Cond B"=w950) -> (w968:T70)
        n493 = call "HEWH Check Power Set.vi"("Station Data Output"=w934, "Timer"=w929, "HEWH Power"=w938) -> ("Set Power To This Value"=w936:bool, "Trigger Power Set"=w937:bool)  [unwired: 6 in, 1 out]
        n494 = case shown="True" w937 {
          tunnel: w936 -> [_ w973]
          frame False {
          }
          frame True {
            n495 = property on="HEWH Power" class="Bool (strict)"("Val(Sgnl)"=w973) -> ()  [unwired: 2 in, 2 out]
            n496 = case shown="True" w973 {
              tunnel: ["Power OFF..." ("Set Status") "Power ON..." ("Set Status")] -> w974
              frame False {
              }
              frame True {
              }
            }
            n497 = call "UTILITY String Notifier.vi"("Status"=UTILITY_Notifier."Set", "Set Status"=w974, "name (unnamed)"="MessageB") -> ()  [unwired: 7 in, 2 out]
          }
        }
        n498 = call <vilib>:"Add State(s) to Queue__jki_lib_state_machine.vi"("State(s) in Front (\"\")"=w962, "State(s) in (\"\")"=w972) -> ("States Out"=w971:string)  [unwired: 13 in]
      }
      frame "Test: Wait for Power Off (Station C)" {
        # "C Timer"
        # "Main Test Loop: Decides which Tank to Run, and starts that sequence."
        n499 = local read "Core HEWH Data Input C"() -> (w1023:T12)
        n500 = Unbundle By Name(w1039) -> ("Station C Display.Display Data (RLT)"=w1030:T29, "Draw Parameters Seq"=w1036:T41, "Current Cond C"=w1022:T1, "Draw Parameters Seq.Station C.Reset Timer"=w996:bool)
        n501 = Bundle By Name(cluster=w1023, "Current Cond"=w1022) -> (w1021:T12)
        n502 = call "HEWH Station Timer.vi"("Station ID"=Station_ID_Selector."C", "error in (no error)"=w995, "Reset Timer (A)"="Reset Timer (C)", "Reset Timer (Cluster)"=w996) -> ("error out"=w1001:errorcluster, "Elapsed Time (sec)- String"=w997:string, "Elapsed Time (sec)"=w999:dbl)  [unwired: 5 in]
        "C Timer" <- w999
        n503 = call "UTILITY String Notifier.vi"("Status"=UTILITY_Notifier."Set", "error in (no error)"=w1001, "Set Status"=w997, "name (unnamed)"="TimerC") -> ("error out"=w1000:errorcluster)  [unwired: 6 in, 1 out]
        n504 = local read "Purge Time (Seconds)"() -> (w998:dbl)
        n505 = local read "Draw Station"() -> (w1028:string)
        n506 = local read "Start Draw"() -> (w1033:bool)
        n507 = Format Date/Time String(time format string (%c)="%H:%M:%S%3u", seconds (now)=w999, UTC format=TRUE) -> (date/time string=→"Timer 3":string)
        n508 = call "HEWH Conditional Trigger.vi"("Draw Parameters Seq"=w1036, "Core HEWH Data Input"=w1021, "Station"="C", "Manual Draw Trigger"="Trigger Draw C", "Draw Station"=w1028, "Error In"=w1000, "Start Draw"=w1033, "Purge Time (sec)"=w998, "Delay After Cutout (sec)"="Cutout Delay C (sec)", "A Timer"=w999, "Disable Station in"="Disable Station 3", "StationA Setpoint"="StationC Setpoint", "Display Data (RLT) In"=w1030) -> ("Station Data Output"=w1004:T14, "Use Last Start Condition?"=→"Use Last Start Condition C?":bool, "SM States"=w1032:string, "Display Data (RLT) Out"=w1029:T29, "Core HEWH Data Output"=w1013:T12, "Disable Station"=w1017:bool, "Error Out"=w1020:errorcluster)  [unwired: 7 in, 1 out]
        n509 = Unbundle By Name(w1013) -> ("Current Cond"=w1018:T1)
        "Condition C" <- w1018
        n510 = Unbundle By Name(w1013) -> ("Test Complete"=w1012:bool)
        "Test CompleteC" <- w1012
        n511 = call "HEWH End Of Test Display.vi"("String Notifier"="MessageC" ("name (unnamed)"), "error in (no error)"=w1020, "Disable Station"=w1017, "Current Cond"=w1018) -> ("error out"=w1015:errorcluster, "Failure"=w1011:bool)  [unwired: 6 in]
        n512 = local read "HEWH Power"() -> (w1007:bool)
        n513 = Or(x=w1011, y=w1017) -> (x .or. y?=w1016:bool)
        n514 = case shown="True" w1016 {
          tunnel: w1015 -> [w1049 w1054]
          tunnel: [w1049 w1053] -> w1014
          tunnel: w1012 -> [_ w1052]
          tunnel: w1011 -> [_ w1050]
          frame False {
          }
          frame True {
            n515 = Or(x=w1052, y=w1050) -> (x .or. y?=w1051:bool)
            n516 = case shown="True" w1051 {
              tunnel: w1054 -> [w1056 w1059]
              tunnel: [w1056 w1058] -> w1053
              frame False {
              }
              frame True {
                n517 = flat-sequence {
                  tunnel: w1059 -> [w1062]
                  tunnel: [w1062] -> w1057
                  tunnel: [w1064] -> w1058
                  tunnel: w1057 -> [w1064]
                  frame #0 {
                    n518 = local write "Log Data Output (C)"(FALSE ("Log Data Output (A)")) -> ()
                    n519 = local write "Station ID to Reset"(Station_ID_Selector."C" ("Station ID to Reset")) -> ()
                  }
                  frame #1 {
                    "Final Headers C" <- TRUE ("Final Headers C")
                  }
                }
              }
            }
            n520 = local write "Disable Station 3"(HEWH_RLT_Station_Disable."Disable Station (No Draw)" ("Disable Station 1")) -> ()
          }
        }
        n521 = call "HEWH Check Power Set.vi"("Station Data Output"=w1004, "Timer"=w999, "HEWH Power"=w1007) -> ("Set Power To This Value"=w1005:bool, "Trigger Power Set"=w1006:bool)  [unwired: 6 in, 1 out]
        n522 = case shown="True" w1006 {
          tunnel: w1005 -> [_ w1043]
          frame False {
          }
          frame True {
            n523 = property on="HEWH Power" class="Bool (strict)"("Val(Sgnl)"=w1043) -> ()  [unwired: 2 in, 2 out]
            n524 = case shown="True" w1043 {
              tunnel: ["Power OFF..." ("Set Status") "Power ON..." ("Set Status")] -> w1044
              frame False {
              }
              frame True {
              }
            }
            n525 = call "UTILITY String Notifier.vi"("Status"=UTILITY_Notifier."Set", "Set Status"=w1044, "name (unnamed)"="MessageC") -> ()  [unwired: 7 in, 2 out]
          }
        }
        n526 = Bundle By Name(cluster=w1039, "Station C Display.Display Data (RLT)"=w1029, "Current Cond C"=w1018) -> (w1038:T70)
        n527 = call <vilib>:"Add State(s) to Queue__jki_lib_state_machine.vi"("State(s) in Front (\"\")"=w1032, "State(s) in (\"\")"=w1042) -> ("States Out"=w1041:string)  [unwired: 13 in]
      }
      frame "Test: Wait for Power Off (Station D)" {
        # "D Timer"
        # "Main Test Loop: Decides which Tank to Run, and starts that sequence."
        n528 = Unbundle By Name(w1109) -> ("Station D Display.Display Data (RLT)"=w1099:T29, "Draw Parameters Seq"=w1106:T41, "Current Cond D"=w1091:T1, "Draw Parameters Seq.Station D.Reset Timer"=w1066:bool)
        n529 = call "HEWH Station Timer.vi"("Station ID"=Station_ID_Selector."D", "error in (no error)"=w1065, "Reset Timer (A)"="Reset Timer (D)", "Reset Timer (Cluster)"=w1066) -> ("error out"=w1071:errorcluster, "Elapsed Time (sec)- String"=w1067:string, "Elapsed Time (sec)"=w1069:dbl)  [unwired: 5 in]
        "D Timer" <- w1069
        n530 = local read "Core HEWH Data Input D"() -> (w1093:T12)
        n531 = local read "Purge Time (Seconds)"() -> (w1068:dbl)
        n532 = Bundle By Name(cluster=w1093, "Current Cond"=w1091) -> (w1092:T12)
        n533 = local read "Draw Station"() -> (w1098:string)
        n534 = local read "Start Draw"() -> (w1103:bool)
        n535 = Format Date/Time String(time format string (%c)="%H:%M:%S%3u", seconds (now)=w1069, UTC format=TRUE) -> (date/time string=→"Timer 4":string)
        n536 = call "UTILITY String Notifier.vi"("Status"=UTILITY_Notifier."Set", "error in (no error)"=w1071, "Set Status"=w1067, "name (unnamed)"="TimerD") -> ("error out"=w1070:errorcluster)  [unwired: 6 in, 1 out]
        n537 = call "HEWH Conditional Trigger.vi"("Draw Parameters Seq"=w1106, "Core HEWH Data Input"=w1092, "Station"="D", "Manual Draw Trigger"="Trigger Draw D", "Draw Station"=w1098, "Error In"=w1070, "Start Draw"=w1103, "Purge Time (sec)"=w1068, "Delay After Cutout (sec)"="Cutout Delay D (sec)", "A Timer"=w1069, "Disable Station in"="Disable Station 4", "StationA Setpoint"="StationD Setpoint", "Display Data (RLT) In"=w1099) -> ("Station Data Output"=w1074:T14, "Use Last Start Condition?"=→"Use Last Start Condition D?":bool, "SM States"=w1102:string, "Display Data (RLT) Out"=w1100:T29, "Core HEWH Data Output"=w1083:T12, "Disable Station"=w1087:bool, "Error Out"=w1090:errorcluster)  [unwired: 7 in, 1 out]
        n538 = Unbundle By Name(w1083) -> ("Current Cond"=w1088:T1)
        "Condition D" <- w1088
        n539 = Unbundle By Name(w1083) -> ("Test Complete"=w1082:bool)
        "Test CompleteD" <- w1082
        n540 = call "HEWH End Of Test Display.vi"("String Notifier"="MessageD" ("name (unnamed)"), "error in (no error)"=w1090, "Disable Station"=w1087, "Current Cond"=w1088) -> ("error out"=w1085:errorcluster, "Failure"=w1081:bool)  [unwired: 6 in]
        n541 = Or(x=w1081, y=w1087) -> (x .or. y?=w1086:bool)
        n542 = Bundle By Name(cluster=w1109, "Station D Display.Display Data (RLT)"=w1100, "Current Cond D"=w1088) -> (w1108:T70)
        n543 = local read "HEWH Power"() -> (w1077:bool)
        n544 = case shown="True" w1086 {
          tunnel: w1085 -> [w1119 w1124]
          tunnel: [w1119 w1123] -> w1084
          tunnel: w1082 -> [_ w1122]
          tunnel: w1081 -> [_ w1120]
          frame False {
          }
          frame True {
            n545 = Or(x=w1122, y=w1120) -> (x .or. y?=w1121:bool)
            n546 = case shown="True" w1121 {
              tunnel: w1124 -> [w1126 w1129]
              tunnel: [w1126 w1128] -> w1123
              frame False {
              }
              frame True {
                n547 = flat-sequence {
                  tunnel: w1129 -> [w1132]
                  tunnel: [w1132] -> w1127
                  tunnel: [w1134] -> w1128
                  tunnel: w1127 -> [w1134]
                  frame #0 {
                    n548 = local write "Log Data Output (D)"(FALSE ("Log Data Output (A)")) -> ()
                    n549 = local write "Station ID to Reset"(Station_ID_Selector."D" ("Station ID to Reset")) -> ()
                  }
                  frame #1 {
                    "Final Headers D" <- TRUE ("Final Headers D")
                  }
                }
              }
            }
            n550 = local write "Disable Station 4"(HEWH_RLT_Station_Disable."Disable Station (No Draw)" ("Disable Station 1")) -> ()
          }
        }
        n551 = call "HEWH Check Power Set.vi"("Station Data Output"=w1074, "Timer"=w1069, "HEWH Power"=w1077) -> ("Set Power To This Value"=w1075:bool, "Trigger Power Set"=w1076:bool)  [unwired: 6 in, 1 out]
        n552 = case shown="True" w1076 {
          tunnel: w1075 -> [_ w1113]
          frame False {
          }
          frame True {
            n553 = property on="HEWH Power" class="Bool (strict)"("Val(Sgnl)"=w1113) -> ()  [unwired: 2 in, 2 out]
            n554 = case shown="True" w1113 {
              tunnel: ["Power OFF..." ("Set Status") "Power ON..." ("Set Status")] -> w1114
              frame False {
              }
              frame True {
              }
            }
            n555 = call "UTILITY String Notifier.vi"("Status"=UTILITY_Notifier."Set", "Set Status"=w1114, "name (unnamed)"="MessageD") -> ()  [unwired: 7 in, 2 out]
          }
        }
        n556 = call <vilib>:"Add State(s) to Queue__jki_lib_state_machine.vi"("State(s) in Front (\"\")"=w1102, "State(s) in (\"\")"=w1112) -> ("States Out"=w1111:string)  [unwired: 13 in]
      }
      frame "Check for UI Event" {
        n557 = local read "Shutdown"() -> (w1139:string)
        n558 = call <vilib>:"Add State(s) to Queue__jki_lib_state_machine.vi"("State(s) in Front (\"\")"=w1139, "State(s) in (\"\")"=w1140) -> ("States Out"=w1138:string)  [unwired: 13 in]
        n559 = flat-sequence {
          tunnel: w1138 -> [w1143]
          tunnel: [w1143] -> w1137
          frame #0 {
            n560 = local write "Shutdown"("" ("Shutdown")) -> ()
          }
        }
        n561 = call <vilib>:"Add State(s) to Queue__jki_lib_state_machine.vi"("State(s) in (\"\")"=w1137) -> ("States Out"=w1142:string)  [unwired: 14 in]
      }
      frame "---------- Main Control ----------" {
        n562 = call <vilib>:"Add State(s) to Queue__jki_lib_state_machine.vi"("State(s) in (\"\")"=w1146) -> ("States Out"=w1149:string)  [unwired: 14 in]
      }
      frame "Temp Decline A" {
        n563 = Unbundle By Name(w1156) -> ("Draw Parameters Seq"=w1151:T41)
        n564 = local read "Temp Decline Complete A"() -> (w1154:bool)
        n565 = call "HEWH Temperature Decline.vi"("Error In"=w1152, "Station"="A", "Temp Decline Complete A"=w1154, "Draw Parameters Seq"=w1151) -> ("Error Out"=w1150:errorcluster, "Output States"=w1155:string)  [unwired: 5 in, 1 out]
        n566 = call <vilib>:"Add State(s) to Queue__jki_lib_state_machine.vi"("State(s) in Front (\"\")"=w1155, "State(s) in (\"\")"=w1159) -> ("States Out"=w1158:string)  [unwired: 13 in]
      }
      frame "Temp Decline B" {
        n567 = Unbundle By Name(w1166) -> ("Draw Parameters Seq"=w1165:T41)
        n568 = local read "Temp Decline Complete B"() -> (w1161:bool)
        n569 = call "HEWH Temperature Decline.vi"("Error In"=w1162, "Station"="B", "Temp Decline Complete A"=w1161, "Draw Parameters Seq"=w1165) -> ("Error Out"=w1160:errorcluster, "Output States"=w1164:string)  [unwired: 5 in, 1 out]
        n570 = call <vilib>:"Add State(s) to Queue__jki_lib_state_machine.vi"("State(s) in Front (\"\")"=w1164, "State(s) in (\"\")"=w1169) -> ("States Out"=w1168:string)  [unwired: 13 in]
      }
      frame "Temp Decline C" {
        n571 = local read "Temp Decline Complete C"() -> (w1171:bool)
        n572 = Unbundle By Name(w1176) -> ("Draw Parameters Seq"=w1175:T41)
        n573 = call "HEWH Temperature Decline.vi"("Error In"=w1172, "Station"="C", "Temp Decline Complete A"=w1171, "Draw Parameters Seq"=w1175) -> ("Error Out"=w1170:errorcluster, "Output States"=w1174:string)  [unwired: 5 in, 1 out]
        n574 = call <vilib>:"Add State(s) to Queue__jki_lib_state_machine.vi"("State(s) in Front (\"\")"=w1174, "State(s) in (\"\")"=w1179) -> ("States Out"=w1178:string)  [unwired: 13 in]
      }
      frame "Temp Decline D" {
        n575 = Unbundle By Name(w1186) -> ("Draw Parameters Seq"=w1185:T41)
